vi "StitchingModeLinear_KJM.vi"(9 "Data In":dbl[][][](array[numeric])) -> (2 "Data Out":dbl[][](array[numeric]))   [LabVIEW 2020]
doc: "Stitches spectra based on simple cut-off modus."
uses:
  6589c867-1e1d-4782-ba12-336f8057cb8d.vi
panel:
  out "deleted portion":dbl[](array[numeric])
  out "subarray":dbl[](array[numeric])
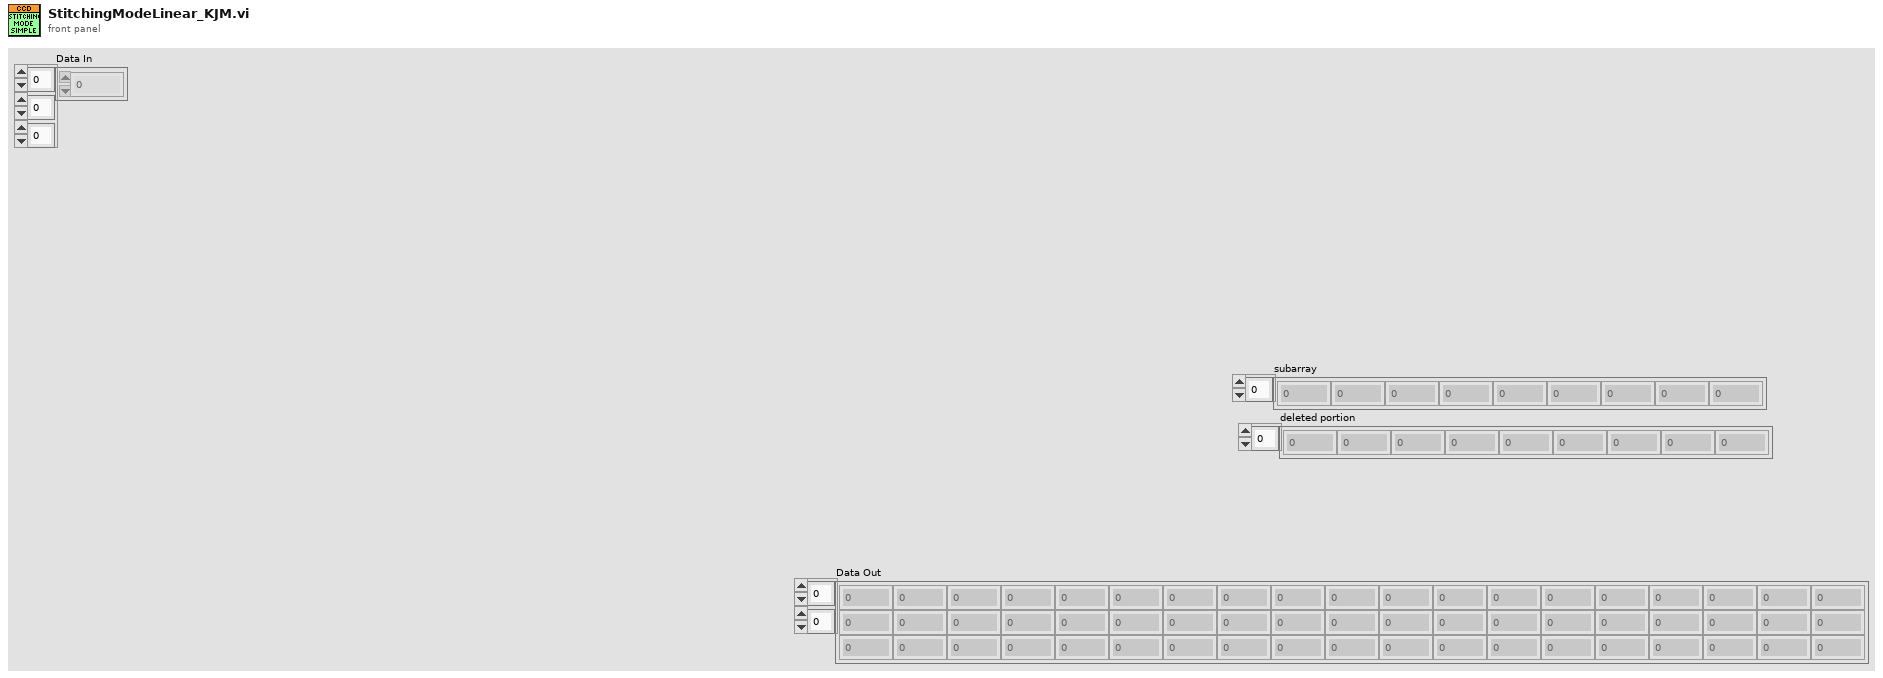
[diagram p1: front panel]
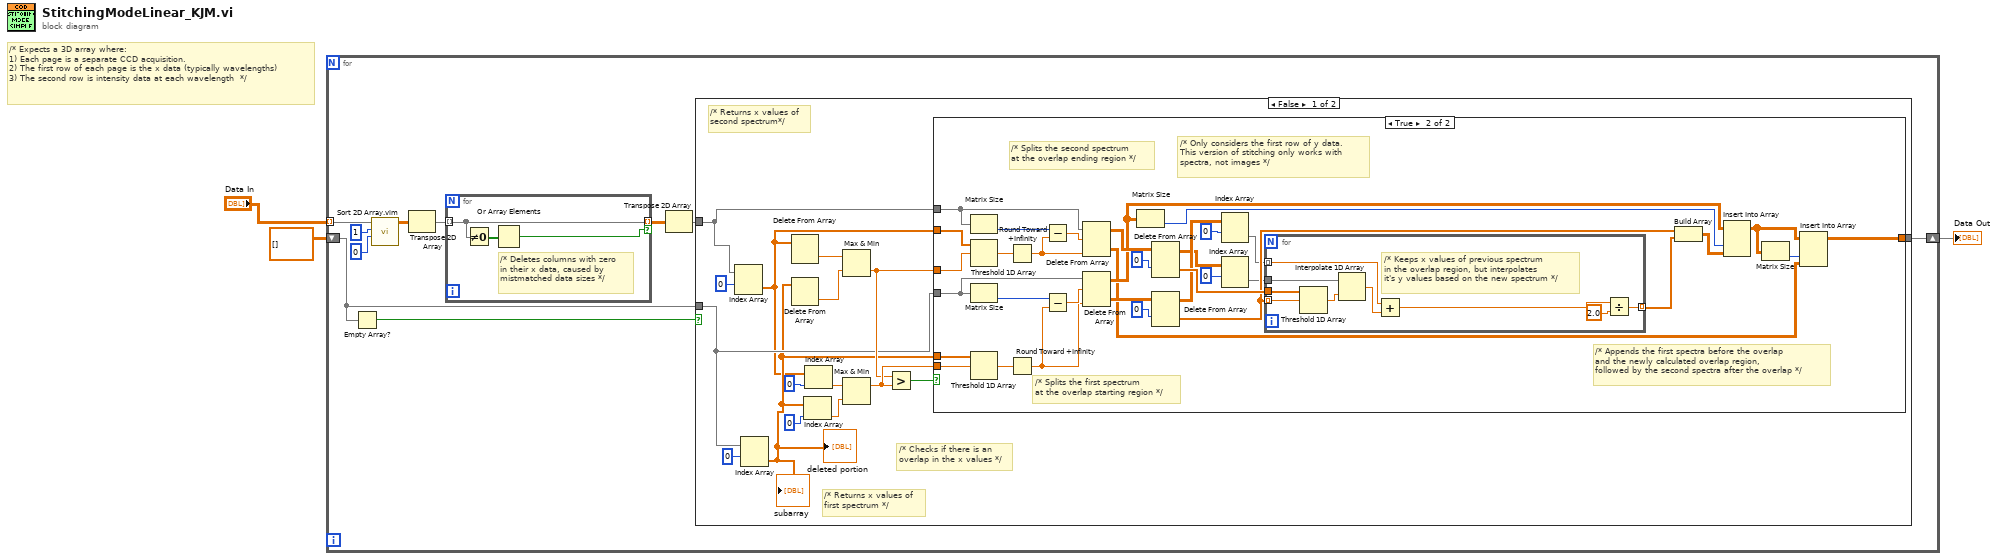
[diagram p0: block diagram]
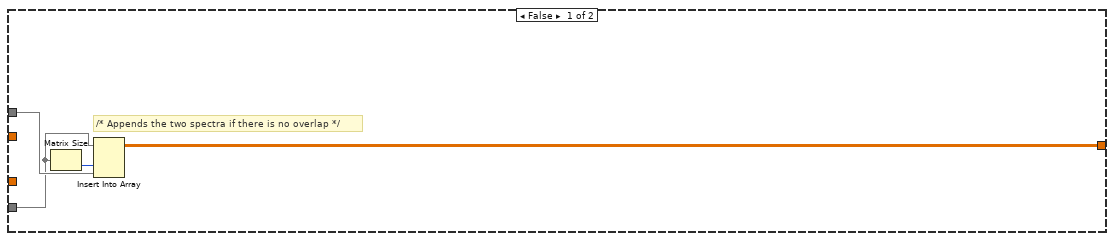
[diagram p2: hidden frame]
diagram:
  # "/* Expects a 3D array where:\n1) Each page is a separate CCD acquisition.\n2) The first row of each page is the x data (typically wavelengths)\n3) The second row is intensity data at each wavelength  */"
  n1 = for {
    tunnel: "Data In" -> [w5] mode=indexing
    shift-right: [w11] -> w2
    shift-left: dbl[][] [] ("Empty Array") -> [w12]
    n2 = Empty Array?(array=w12) -> (empty?=w13:bool)
    n3 = call "Sort 2D Array.vim"("index"=0, "dimension to index (column)"=1 ("index"), "2D array"=w5) -> ("sorted 2D array"=w6:dbl[][])  [unwired: 7 in, 1 out]
    n4 = Transpose 2D Array(2D array=w6) -> (transposed array=w10:dbl[][])
    n5 = for {
      tunnel: w10 -> [w15] mode=indexing
      tunnel: [w15] -> w9 mode=indexing if=w16
      # "/* Deletes columns with zero\nin their x data, caused by\nmistmatched data sizes */"
      n6 = Not Equal To 0?(x=w15) -> (x != 0?=w14:bool[])
      n7 = Or Array Elements(Boolean array=w14) -> (logical OR=w16:bool)
    }
    n8 = Transpose 2D Array(2D array=w9) -> (transposed array=w4:dbl[][])
    n9 = case shown="False" w13 {
      tunnel: w12 -> [w22 _]
      tunnel: w4 -> [w18 w80]
      tunnel: [w23 w80] -> w11
      frame False {
        # "/* Checks if there is an \noverlap in the x values */"
        # "/* Returns x values of \nfirst spectrum */"
        # "/* Returns x values of \nsecond spectrum*/"
        n10 = Index Array(array=w18, index (row)=0) -> (element=w17:dbl[])  [unwired: 1 in]
        n11 = Index Array(array=w22, index (row)=0) -> (element=w20:dbl[])  [unwired: 1 in]
        "subarray" <- w20
        "deleted portion" <- w20
        n12 = Delete From Array(array=w17) -> (deleted portion=w28:dbl)  [unwired: 2 in, 1 out]
        n13 = Delete From Array(array=w20) -> (deleted portion=w27:dbl)  [unwired: 2 in, 1 out]
        n14 = Index Array(array=w20, index=0) -> (element=w29:dbl)
        n15 = Index Array(array=w17, index=0) -> (element=w30:dbl)
        n16 = Max & Min(x=w28, y=w27) -> (min(x,y)=w24:dbl)  [unwired: 1 out]
        n17 = Max & Min(x=w30, y=w29) -> (max(x,y)=w25:dbl)  [unwired: 1 out]
        n18 = Greater?(x=w24, y=w25) -> (0:w26:bool)
        n19 = case shown="True" w26 {
          tunnel: w25 -> [_ w55]
          tunnel: w24 -> [_ w58]
          tunnel: w17 -> [_ w59]
          tunnel: w18 -> [w35 w60]
          tunnel: w22 -> [w34 w57]
          tunnel: w20 -> [_ w56]
          tunnel: [w33 w43] -> w23
          frame False {
            # "/* Appends the two spectra if there is no overlap */"
            n20 = Matrix Size(0:w34) -> (2:w36:i32)  [unwired: 1 out]
            n21 = Insert Into Array(array=w34, index (col)=w36, new element=w35) -> (w33:dbl[][])  [unwired: 1 in]
          }
          frame True {
            # "/* Only considers the first row of y data. \nThis version of stitching only works with \nspectra, not images */"
            # "/* Splits the second spectrum \nat the overlap ending region */"
            # "/* Splits the first spectrum \nat the overlap starting region */"
            # "/* Appends the first spectra before the overlap\nand the newly calculated overlap region, \nfollowed by the second spectra after the overlap */"
            n22 = Matrix Size(0:w60) -> (2:w65:i32)  [unwired: 1 out]
            n23 = Threshold 1D Array(2:w58, 3:w59) -> (0:w66:dbl)  [unwired: 1 in]
            n24 = Matrix Size(0:w57) -> (2:w69:i32)  [unwired: 1 out]
            n25 = Threshold 1D Array(2:w55, 3:w56) -> (0:w70:dbl)  [unwired: 1 in]
            n26 = Round Toward +Infinity(x=w66) -> (ceil(x): smallest int >= x=w63:dbl)
            n27 = Round Toward +Infinity(x=w70) -> (ceil(x): smallest int >= x=w67:dbl)
            n28 = Subtract(x=w65, y=w63) -> (x-y=w64:dbl)
            n29 = Subtract(x=w69, y=w67) -> (x-y=w68:dbl)
            n30 = Delete From Array(array=w60, length=w64, index (col)=w63) -> (deleted portion=w44:dbl[][], array with subset deleted=w53:dbl[][])  [unwired: 1 in]
            n31 = Delete From Array(array=w57, length=w68, index (col)=w67) -> (deleted portion=w62:dbl[][], array with subset deleted=w50:dbl[][])  [unwired: 1 in]
            n32 = Matrix Size(0:w50) -> (2:w51:i32)  [unwired: 1 out]
            n33 = Delete From Array(array=w53, index (row)=0) -> (deleted portion=w52:dbl[], array with subset deleted=w39:dbl[][])  [unwired: 2 in]
            n34 = Delete From Array(array=w62, index (row)=0) -> (deleted portion=w49:dbl[], array with subset deleted=w42:dbl[][])  [unwired: 2 in]
            n35 = Index Array(array=w42, index (row)=0) -> (element=w40:dbl[])  [unwired: 1 in]
            n36 = Index Array(array=w39, index (row)=0) -> (element=w38:dbl[])  [unwired: 1 in]
            n37 = for {
              tunnel: w52 -> [w78]
              tunnel: w49 -> [w76] mode=indexing
              tunnel: [w73] -> w48 mode=indexing
              tunnel: w38 -> [w71]
              tunnel: w40 -> [w72] mode=indexing
              # "/* Keeps x values of previous spectrum\nin the overlap region, but interpolates \nit's y values based on the new spectrum */"
              n38 = Threshold 1D Array(2:w76, 3:w78) -> (0:w79:dbl)  [unwired: 1 in]
              n39 = Interpolate 1D Array(1:w79, 2:w71) -> (0:w77:dbl)
              n40 = Add(x=w72, y=w77) -> (x+y=w75:dbl)
              n41 = Divide(x=w75, y=2.0) -> (x/y=w73:dbl)
            }
            n42 = Build Array(w49, w48) -> (w47:dbl[][])
            n43 = Insert Into Array(array=w50, index (col)=w51, new element=w47) -> (w46:dbl[][])  [unwired: 1 in]
            n44 = Matrix Size(0:w46) -> (2:w45:i32)  [unwired: 1 out]
            n45 = Insert Into Array(array=w46, index (col)=w45, new element=w44) -> (w43:dbl[][])  [unwired: 1 in]
          }
        }
      }
      frame True {
        # "/* Runs on the first loop only, and returns the spectrum */"
      }
    }
  }
  "Data Out" <- w2
